vi "Clamp Until Held, Then Lift.vi"(1 "Iterations":i32=1, 2 "Clamp + Lift":bool) -> ()   [LabVIEW 2014]
uses:
  Precreated VIs/Robot Global Data.vi
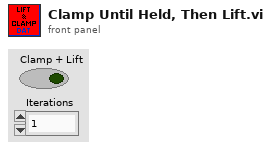
[diagram p1: front panel]
types:
  T1 = cluster{"Pickup Mechanism":cluster{"Lift":cluster{"Top":bool, "High":bool, "Mid":bool, "Low":bool, "Bot":bool}, "Clamp":cluster{"Widest":bool, "Shortest":bool, "Tote 1":bool, "Tote 2":bool}}, "Ultrasonic":dbl, "Clamper Wide":bool, "Tote in?":bool, "Liff Encoder":dbl}
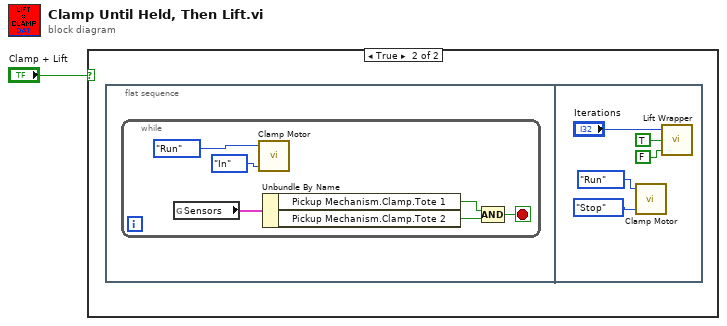
[diagram p0: block diagram]
diagram:
  n1 = case shown="True" "Clamp + Lift" {
    frame False {
    }
    frame True {
      n2 = flat-sequence {
        frame #0 {
          n3 = while {
            stop <- w2 stop-if-true
            n4 = global read "Robot Global Data.vi" "Sensors"() -> (w5:T1)
            n5 = call "Clamp Motor.vi"("Direction"=enum16{"Stop", "In", "Out"}."In", "Mode"=enum8{"Start", "Run", "Finish"}."Run") -> ()  [unwired: 1 in]
            n6 = Unbundle By Name(w5) -> ("Pickup Mechanism.Clamp.Tote 1"=w4:bool, "Pickup Mechanism.Clamp.Tote 2"=w3:bool)
            n7 = Compound Arithmetic op=AND(w4, w3) -> (w2:bool)
          }
        }
        frame #1 {
          n8 = call "Clamp Motor.vi"("Direction"=enum16{"Stop", "In", "Out"}."Stop", "Mode"=enum8{"Start", "Run", "Finish"}."Run") -> ()  [unwired: 1 in]
          n9 = call "Lift Wrapper.vi"("Down"=FALSE ("Up or Down"), "Up"=TRUE ("Up or Down"), "Iterations"="Iterations") -> ()
        }
      }
    }
  }
